vi "Sub_Labview_eigh.vi"(2 "Mass":T2=array398x398[158404 elements], 3 "Stiffness":T2=array398x398[158404 elements]) -> (0 "Eigenvectors":T1, 1 "Eigenvalues":cdb[](array[numeric])=[2.2804432673463e+16+0.0i, 2.2791801241660108e+16+0.0i, 2.2770775777903908e+16+0.0i, 2.2741396645419244e+16+0.0i, 2.270371987785269e+16+0.0i, 2.2657817239183124e+16+0.0i, 2.2603775716234956e+16+0.0i, 2.254169702884662e+16+0.0i, 2.2471697376480412e+16+0.0i, 2.2393906855337016e+16+0.0i, 2.230846857910318e+16+0.0i, 2.221553847521475e+16+0.0i, 2.2115284355411816e+16+0.0i, 2.2007885236471344e+16+0.0i, 2.189353050374903e+16+0.0i, 2.1772419242137296e+16+0.0i, 2.164475925432977e+16+0.0i, 2.1510766589189344e+16+0.0i, 2.1370664150481036e+16+0.0i, 2.122468133385367e+16+0.0i, 2.10730528717859e+16+0.0i, 2.091601815021323e+16+0.0i, 2.0753820215894624e+16+0.0i, 2.0586705176648892e+16+0.0i, 2.0414921126128804e+16+0.0i, 2.0238717520685452e+16+0.0i, 2.0058344603829756e+16+0.0i, 1.9874052173444412e+16+0.0i, 1.96860893461687e+16+0.0i, 1.9494703748234612e+16+0.0i, 1.9300140832028e+16+0.0i, 1.910264334910452e+16+0.0i, 1.8902450850069396e+16+0.0i, 1.869979902209041e+16+0.0i, 1.849491946531884e+16+0.0i, 1.828803903285659e+16+0.0i, 1.807937953400631e+16+0.0i, 1.786915748292412e+16+0.0i, 1.7657583633898862e+16+0.0i, 1.7444862864139334e+16+0.0i, 1.7231193829226492e+16+0.0i, 1.7016768880520596e+16+0.0i, 1.680177378317798e+16+0.0i, 1.6586387752006862e+16+0.0i, 1.6370783114606408e+16+0.0i, 1.6155125634801468e+16+0.0i, 1.5939574000401302e+16+0.0i, 1.5724280227036932e+16+0.0i, 1.550938942058045e+16+0.0i, 1.5295039933221446e+16+0.0i, 1.5081363358574598e+16+0.0i, 1.4868484707567944e+16+0.0i, 1.465652230809223e+16+0.0i, 1.444558816577803e+16+0.0i, 1.4235787888765144e+16+0.0i, 1.4027220917039866e+16+0.0i, 1.3819980579927174e+16+0.0i, 1.3614154409670614e+16+0.0i, 1.3409824100383668e+16+0.0i, 1.3207065816981184e+16+0.0i, 1.300595034102125e+16+0.0i, 1.2806543231097902e+16+0.0i, 1.260890496424712e+16+0.0i, 1.2413091157942396e+16+0.0i, 1.2219152761289788e+16+0.0i, 1.2027136247875668e+16+0.0i, 1.1837083736591752e+16+0.0i, 1.1649033184678588e+16+0.0i, 1.1463018676336632e+16+0.0i, 1.127907039239082e+16+0.0i, 1.109721502126191e+16+0.0i, 1.0917475693677812e+16+0.0i, 1.0739872348790558e+16+0.0i, 1.0564421769754534e+16+0.0i, 1.0391137844680336e+16+0.0i, 1.0220031564066164e+16+0.0i, 1.0051111375992904e+16+0.0i, 9884383166941636.0+0.0i, 9719850434335504.0+0.0i, 9557514519724968.0+0.0i, 9397374623096130.0+0.0i, 9239428002705814.0+0.0i, 9083670049729966.0+0.0i, 8930094418013950.0+0.0i, 8778693177437564.0+0.0i, 8629456861392506.0+0.0i, 8482374622991416.0+0.0i, 8337434242455708.0+0.0i, 8194622371288402.0+0.0i, 8053924481767733.0+0.0i, 7915325036692032.0+0.0i, 7778807495332094.0+0.0i, 7644354500461822.0+0.0i, 7511947848772199.0+0.0i, 7381568621883960.0+0.0i, 7253197219567342.0+0.0i, 7126813462759133.0+0.0i, 7002396594936877.0+0.0i, 6879925407135902.0+0.0i, 6759378238496308.0+0.0i, 6640733083830347.0+0.0i, 6523967566492697.0+0.0i, 6409059065152816.0+0.0i, 6295984688289724.0+0.0i, 6184721388627444.0+0.0i, 6075245924618110.0+0.0i, 5967534973674746.0+0.0i, 5861565112298633.0+0.0i, 5757312872953094.0+0.0i, 5654754763902227.0+0.0i, 5553867318557252.0+0.0i, 5454627101037715.0+0.0i, 5357010757898036.0+0.0i, 5260995018741689.0+0.0i, 5166556710025747.0+0.0i, 5073672824628966.0+0.0i, 4982320474716886.0+0.0i, 4892476974485616.0+0.0i, 4804119794497124.0+0.0i, 4717226623097733.0+0.0i, 4631775350664416.0+0.0i, 4547744102297698.0+0.0i, 4465111224072673.0+0.0i, 4383855312095715.5+0.0i, 4303955202212639.0+0.0i, 4225389990004321.5+0.0i, 4148139032673850.5+0.0i, 4072181948136458.5+0.0i, 3997498619309947.0+0.0i, 3924069197675197.0+0.0i, 3851874110868095.5+0.0i, 3780894050780673.0+0.0i, 3711109985247617.0+0.0i, 3642503150532603.5+0.0i, 3575055058991141.5+0.0i, 3508747489513928.0+0.0i, 3443562484473190.5+0.0i, 3379482366333986.5+0.0i, 3316489717268121.5+0.0i, 3254567377770020.0+0.0i, 3193698455472225.5+0.0i, 3133866320115410.0+0.0i, 3075054600401521.0+0.0i, 3017247172346058.0+0.0i, 2960428176599958.0+0.0i, 2904582000884634.5+0.0i, 2849693283122604.5+0.0i, 2795746909521275.5+0.0i, 2742728014198788.5+0.0i, 2690621980195449.0+0.0i, 2639414425741431.5+0.0i, 2589091223110994.0+0.0i, 2539638477752609.5+0.0i, 2491042538145654.5+0.0i, 2443289994506425.0+0.0i, 2396367679858359.0+0.0i, 2350262662104751.5+0.0i, 2304962257802260.0+0.0i, 2260454022921744.0+0.0i, 2216725756001909.2+0.0i, 2173765511769162.8+0.0i, 2131561584710583.0+0.0i, 2090102534312290.5+0.0i, 2049377179154158.2+0.0i, 2009374606593172.2+0.0i, 1970084181188089.0+0.0i, 1931495560617783.8+0.0i, 1893598703140482.5+0.0i, 1856383893949433.0+0.0i, 1819841754513909.2+0.0i, 1783963284443140.0+0.0i, 1748739881364360.0+0.0i, 1714163389761557.8+0.0i, 1680226148424105.5+0.0i, 1646921060537150.2+0.0i, 1614241668685292.0+0.0i, 1582182257998151.8+0.0i, 1550737994761724.8+0.0i, 1519905082534945.5+0.0i, 1489680993950089.8+0.0i, 1460064746546831.5+0.0i, 1431057286622201.2+0.0i, 1402661989863789.2+0.0i, 1374885348788757.8+0.0i, 1347737903117768.5+0.0i, 1321235544252224.0+0.0i, 1295401343138600.0+0.0i, 1270268168089524.2+0.0i, 1245882489699087.8+0.0i, 1222309967457149.8+0.0i, 1199643793566512.8+0.0i, 1178017168747350.5+0.0i, 1157621907777862.0+0.0i, 1138735358718552.5+0.0i, 1121756328301595.8+0.0i, 1107243458087227.0+0.0i, 1095929339913804.2+0.0i, 1088649957669511.5+0.0i, 909937758009993.9+0.0i, 891910721202564.9+0.0i, 884934454759382.6+0.0i, 874723979810274.4+0.0i, 862285094163182.1+0.0i, 848355989909978.5+0.0i, 833458094327715.1+0.0i, 817952685669791.2+0.0i, 802088806916336.8+0.0i, 786038959565398.6+0.0i, 769923840620793.5+0.0i, 753828924314225.6+0.0i, 737815465900471.9+0.0i, 721927829689407.6+0.0i, 706198414871018.5+0.0i, 690651013328068.8+0.0i, 675303132784373.4+0.0i, 660167626918822.2+0.0i, 645253859540316.9+0.0i, 630568543874100.6+0.0i, 616116360605280.6+0.0i, 601900415114552.5+0.0i, 587922580396813.2+0.0i, 574183760327140.4+0.0i, 560684088738315.8+0.0i, 547423085293601.1+0.0i, 534399778013495.8+0.0i, 521612798188417.4+0.0i, 509060457743455.1+0.0i, 496740809491096.75+0.0i, 484651696941848.0+0.0i, 472790794899573.8+0.0i, 461155641179870.3+0.0i, 449743664146515.0+0.0i, 438552204727703.7+0.0i, 427578534875682.75+0.0i, 416819872989033.06+0.0i, 406273396574390.25+0.0i, 395936253310089.2+0.0i, 385805570055176.7+0.0i, 375878460267907.06+0.0i, 366152031059008.56+0.0i, 356623388410250.94+0.0i, 347289641907544.4+0.0i, 338147908909055.6+0.0i, 329195317731802.3+0.0i, 320429011027087.4+0.0i, 311846147750000.3+0.0i, 303443905837277.0+0.0i, 295219483465438.3+0.0i, 287170101163036.5+0.0i, 279293002803623.84+0.0i, 271585456633238.9+0.0i, 264044756509003.9+0.0i, 256668222541015.97+0.0i, 249453201536901.44+0.0i, 242397067968510.94+0.0i, 235497223932908.28+0.0i, 228751099707482.3+0.0i, 222156154069208.78+0.0i, 215709874304784.66+0.0i, 209409776517619.72+0.0i, 203253405444754.75+0.0i, 197238334788276.12+0.0i, 191362166857426.9+0.0i, 185622532792031.34+0.0i, 180017092335585.28+0.0i, 174543533707346.38+0.0i, 169199573475812.34+0.0i, 163982956480768.84+0.0i, 158891455479439.34+0.0i, 153922871075542.84+0.0i, 149075031433285.25+0.0i, 144345792100433.72+0.0i, 139733035655498.38+0.0i, 135234671689682.58+0.0i, 130848636244115.92+0.0i, 126572891821172.61+0.0i, 122405426997758.4+0.0i, 118344256036173.22+0.0i, 114387418849248.23+0.0i, 110532980612702.23+0.0i, 106779031382507.62+0.0i, 103123685940825.9+0.0i, 99565083564223.05+0.0i, 96101387581216.72+0.0i, 92730785139576.97+0.0i, 89451487044580.45+0.0i, 86261727362292.8+0.0i, 83159763143655.97+0.0i, 80143874223014.53+0.0i, 77212362869927.75+0.0i, 74363553605060.06+0.0i, 71595792781124.61+0.0i, 68907448494118.57+0.0i, 66296910106615.64+0.0i, 63762588237758.92+0.0i, 61302914288499.9+0.0i, 58916340277289.164+0.0i, 56601338536617.86+0.0i, 54356401488425.04+0.0i, 52180041323067.2+0.0i, 50070789813727.125+0.0i, 48027198000868.24+0.0i, 46047835996272.5+0.0i, 44131292583528.08+0.0i, 42276175110607.94+0.0i, 40481109134113.02+0.0i, 38744738172156.125+0.0i, 37065723428079.62+0.0i, 35442743543535.75+0.0i, 33874494307453.61+0.0i, 32359688389607.785+0.0i, 30897055118985.55+0.0i, 29485340132701.55+0.0i, 28123305260617.945+0.0i, 26809728151436.02+0.0i, 25543402207235.453+0.0i, 24323136280774.438+0.0i, 23147754605824.973+0.0i, 22016096680017.48+0.0i, 20927017174127.316+0.0i, 19879386048501.082+0.0i, 18872088515772.46+0.0i, 17904025312459.027+0.0i, 16974112875378.494+0.0i, 16081283685922.305+0.0i, 15224486657077.748+0.0i, 14402687594584.03+0.0i, 13614869658614.9+0.0i, 12860033905237.787+0.0i, 12137199736136.256+0.0i, 11445405362881.02+0.0i, 10783708168112.809+0.0i, 10151184976956.836+0.0i, 9546932183309.566+0.0i, 8970065740329.162+0.0i, 8419721022281.91+0.0i, 7895052518633.381+0.0i, 7395233418375.991+0.0i, 6919455109633.198+0.0i, 6466926533285.593+0.0i, 6036873586904.214+0.0i, 5628538423739.423+0.0i, 5241178814916.885+0.0i, 4874067513276.024+0.0i, 4526491651970.804+0.0i, 4197752261882.221+0.0i, 3887163785997.987+0.0i, 3594053718336.367+0.0i, 3317762272596.151+0.0i, 3057642138480.3125+0.0i, 2813058314874.0273+0.0i, 2583387949314.072+0.0i, 2368020279576.7393+0.0i, 2166356563521.263+0.0i, 1977810088703.2822+0.0i, 1801806169115.9978+0.0i, 1637782190349.3826+0.0i, 1485187656790.9333+0.0i, 1343484252719.8376+0.0i, 1212145906834.1458+0.0i, 1090658872603.2037+0.0i, 978521802056.0394+0.0i, 875245824616.3925+0.0i, 780354619231.5298+0.0i, 693384492440.8652+0.0i, 613884450915.5371+0.0i, 541416269080.44867+0.0i, 475554556190.9326+0.0i, 415886816618.86835+0.0i, 362013512558.3495+0.0i, 313548113007.63965+0.0i, 270117150347.5564+0.0i, 231360266083.93283+0.0i, 196930257577.8631+0.0i, 166493117567.83093+0.0i, 139728073712.95016+0.0i, 116327626980.8429+0.0i, 95997581988.6117+0.0i, 78457079813.79535+0.0i, 63438626980.45474+0.0i, 50688121841.734344+0.0i, 39964879816.702194+0.0i, 31041656469.031185+0.0i, 23704669002.43506+0.0i, 17753614901.423603+0.0i, 13001692027.533115+0.0i, 9275613725.040789+0.0i, 6415624969.193008+0.0i, 4275515279.325833+0.0i, 2722632472.8846316+0.0i, 1637891666.3815625+0.0i, 915784527.7517059+0.0i, 464384954.46519357+0.0i, 205349469.9890637+0.0i, 73907396.15765077+0.0i, 18842923.72259714+0.0i, 2340326.773945595+0.0i, 57324.18969647021+0.0i] format="%.2f")   [LabVIEW 2021]
uses:
  <vilib>/Analysis/Matrix/Datatypes/RealMatrix.ctl
  <vilib>/Analysis/Matrix/Datatypes/ComplexMatrix.ctl
  <vilib>/Analysis/7linalg.llb/Real Generalized Eigenvalues and Vectors.vi
  <vilib>/Analysis/7linalg.llb/Complex Conjugate Transpose Matrix.vi
  <vilib>/Analysis/baseanly.llb/Complex A x B.vi
  <vilib>/Analysis/Matrix/Numeric/Square Root/Square Root - CM.vi
  <vilib>/Analysis/NI_AALPro.lvlib
  <vilib>/Analysis/Matrix/NI_Matrix.lvlib
  <vilib>/Analysis/NI_AALBase.lvlib
panel:
  out "error out":errorcluster
  # "Documentation\n\nLorem Ipsum"
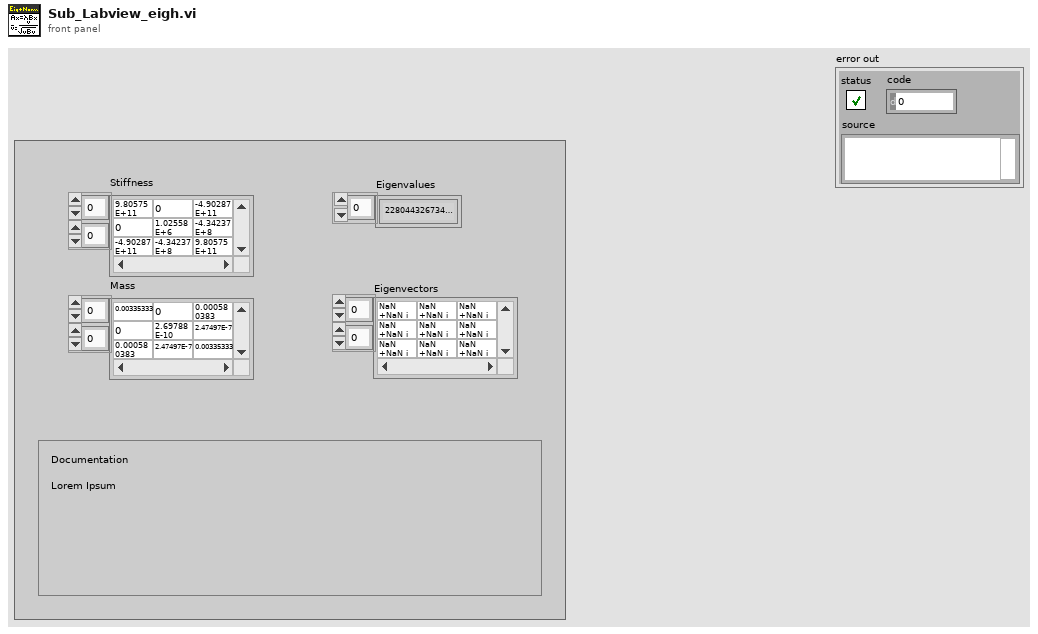
[diagram p1: front panel]
types:
  T1 = typedef "NI_Matrix.lvlib/ComplexMatrix.ctl" = cdb[][]
  T2 = typedef "NI_Matrix.lvlib/RealMatrix.ctl" = dbl[][]
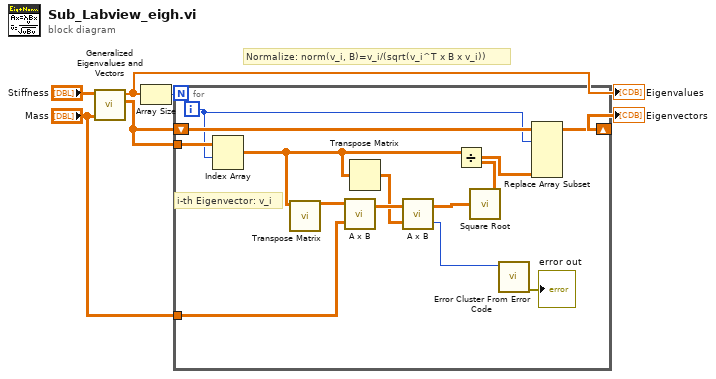
[diagram p0: block diagram]
diagram:
  # "Normalize: norm(v_i, B)=v_i/(sqrt(v_i^T x B x v_i))"
  n1 = call-poly <vilib>:"Generalized Eigenvalues and Vectors.vi"("B"="Mass", "A"="Stiffness") -> ("Eigenvectors"=w2:T1, "Eigenvalues"=w6:cdb[])  [unwired: 4 in, 1 out]
  "Eigenvalues" <- w6
  n2 = Array Size(array=w6) -> (size(s)=w3:i32)
  n3 = for {
    N: w3 -> [_]
    tunnel: w2 -> [w20]
    tunnel: "Mass" -> [w19]
    shift-right: [w15] -> w1
    shift-left: w2 -> [w16]
    i -> [w14]
    # "i-th Eigenvector: v_i"
    n4 = Index Array(array=w20, index (row)=w14) -> (element=w11:T1)  [unwired: 1 in]
    n5 = call-poly <vilib>:"Transpose Matrix.vi"("Input Matrix"=w11) -> ("Matrix Conjugate Transpose"=w13:T1)  [unwired: 9 in, 1 out]
    n6 = call-poly <vilib>:"A x B.vi"("B"=w19, "A"=w13) -> ("A x B"=w10:T1)  [unwired: 1 out]
    n7 = Transpose Matrix(1:w11) -> (0:w9:T1)
    n8 = call-poly <vilib>:"A x B.vi"("B"=w9, "A"=w10) -> ("error"=w8:i32, "A x B"=w18:T1)
    n9 = call-poly <vilib>:"Square Root.vi"("Complex Matrix A"=w18) -> ("sqrt(A)"=w17:T1)
    n10 = Divide(x=w11, y=w17) -> (x/y=w12:T1)
    n11 = call <vilib>:"Error Cluster From Error Code.vi"("error code (0)"=w8) -> ("error out"=→"error out":errorcluster)  [unwired: 8 in]
    n12 = Replace Array Subset(array=w16, new element=w12, index (dim 0)=w14) -> (w15:T1)  [unwired: 3 in]
  }
  "Eigenvectors" <- w1
